vi "software_roi.vi"(1 "Cut image?":bool, 2 "Input Array":sgl[][](array[numeric])=[[1.0, 2.0, 3.0, 4.0, 5.0, 6.0], [7.0, 8.0, 9.0, 10.0, 11.0, 12.0], [13.0, 14.0, 15.0, 16.0, 17.0, 18.0], [19.0, 20.0, 21.0, 22.0, 23.0, 2.0], [25.0, 26.0, 27.0, 8.0, 29.0, 3.0], [31.0, 2.0, 33.0, 4.0, 35.0, 36.0]], 3 "ROI Controls":T1={"y start"=0, "y stop"=6, "x start"=0, "x stop"=6}) -> (0 "output array":sgl[][](array[numeric]))   [LabVIEW 2013]
panel:
  out "size(s)":i32[](array[numeric])
  out "Cut Image":sgl[][](graph)
  out "Uncut Image":sgl[][](graph)
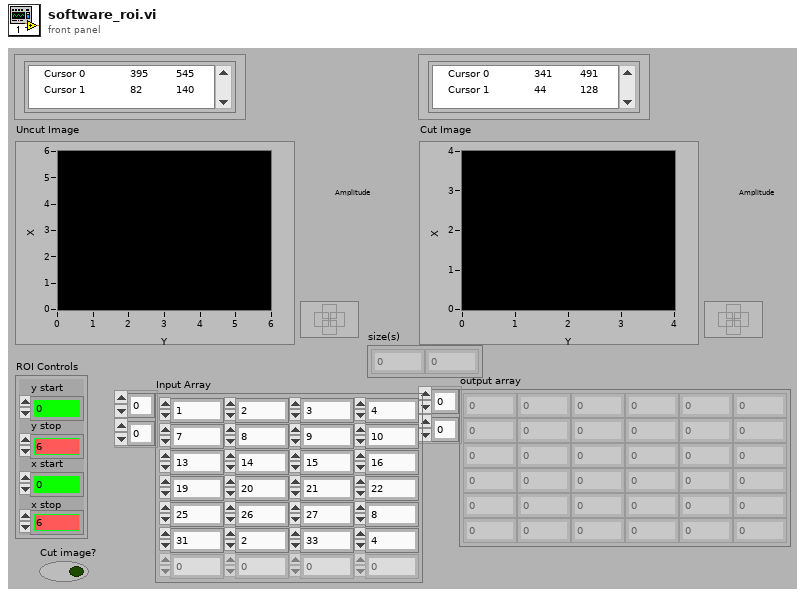
[diagram p1: front panel]
types:
  T1 = cluster{"y start":i32, "y stop":i32, "x start":i32, "x stop":i32}
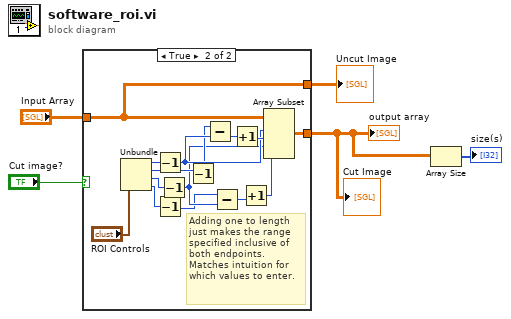
[diagram p0: block diagram]
diagram:
  n1 = case shown="True" "Cut image?" {
    tunnel: "Input Array" -> [w6 w19]
    tunnel: [w6 w21] -> w2
    tunnel: [w6 w19] -> w3
    frame False {
    }
    frame True {
      # "Adding one to length\njust makes the range\nspecified inclusive of\nboth endpoints.\nMatches intuition for\nwhich values to enter."
      n2 = Unbundle("ROI Controls") -> ("y start"=w14:i32, "y stop"=w12:i32, "x start"=w10:i32, "x stop"=w8:i32)
      n3 = Decrement(x=w14) -> (x-1=w13:i32)
      n4 = Decrement(x=w8) -> (x-1=w7:i32)
      n5 = Decrement(x=w10) -> (x-1=w9:i32)
      n6 = Decrement(x=w12) -> (x-1=w11:i32)
      n7 = Subtract(x=w11, y=w13) -> (x-y=w18:i32)
      n8 = Subtract(x=w7, y=w9) -> (x-y=w17:i32)
      n9 = Increment(x=w18) -> (x+1=w15:i32)
      n10 = Increment(x=w17) -> (x+1=w16:i32)
      n11 = Array Subset(array=w19, index (row)=w13, length (row)=w15, index (col)=w9, length (col)=w16) -> (w21:sgl[][])
    }
  }
  "output array" <- w2
  "Cut Image" <- w2
  "Uncut Image" <- w3
  n12 = Array Size(array=w2) -> (size(s)=→"size(s)":i32[])
